vi "Test ESA functionality.vi"   [LabVIEW 2020, in "SA-ESA.lvclass"]
uses:
  SA-ESA.lvclass
  C:/Sandbox/RF Bench/Source Code/WiSpry Test Framework/Instruments/Instrument.lvclass
  Instrument.lvclass/Instrument.ctl
  Instrument.lvclass
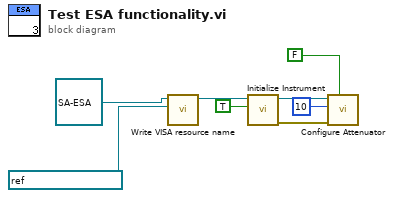
[diagram p0: block diagram]
diagram:
  n1 = call "Write VISA resource name.vi"("VISA resource name"=refnum<visa-resource-name> "GPIB0::18::INSTR", "Instrument in"=refnum<class "SA-ESA.lvclass"> refnum ("SA-ESA.lvclass")) -> ("Instrument out"=w6:refnum<class "SA-ESA.lvclass">)  [unwired: 9 in]
  n2 = call-dynamic "Initialize Instrument.vi"("Reset"=TRUE, "SA-ESA in"=w6) -> ("error out"=w4:errorcluster, "SA-ESA out"=w3:refnum<class "SA-ESA.lvclass">)  [unwired: 8 in]
  n3 = call-dynamic "Configure Attenuator.vi"("Auto Attenuator (T)"=FALSE, "error in (no error)"=w4, "Attenuator (dB)"=u32 10, "SA-ESA in"=w3) -> ()  [unwired: 6 in, 2 out]
